vi "Leja Order Roots.vi"   [LabVIEW 2012, in "NI_AALPro.lvlib"]
uses:
  NI_AALPro.lvlib
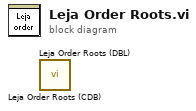
[diagram p0: block diagram]
diagram:
  n1 = call "Leja Order Roots (CDB).vi"() -> ()  [unwired: 11 in, 1 out]
  n2 = call "Leja Order Roots (DBL).vi"() -> ()  [unwired: 11 in, 1 out]
